vi "在image画线.vi"(10 "Image":T1, 11 "一维数组":dbl[](array[numeric])) -> (2 "Image Out":T1)   [LabVIEW 2015]
uses:
  <vilib>/vision/Image Controls.llb/IMAQ Image.ctl
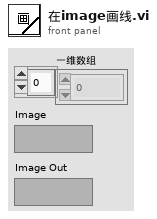
[diagram p1: front panel]
types:
  T1 = typedef "IMAQ Image.ctl" = refnum<image>
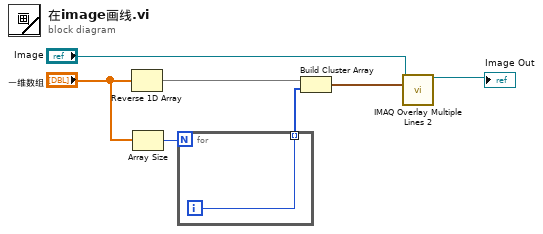
[diagram p0: block diagram]
diagram:
  n1 = Reverse 1D Array(array="一维数组") -> (reversed array=w1:dbl[])
  n2 = Array Size(array="一维数组") -> (size(s)=w6:i32)
  n3 = for {
    N: w6 -> [_]
    tunnel: [w8] -> w7 mode=indexing
    i -> [w8]
  }
  n4 = Build Cluster Array(w1, w7) -> (w5:cluster{"Numeric":dbl, i32}[])
  n5 = call "IMAQ Overlay Multiple Lines 2"("Image"="Image", "Line End Points"=w5) -> ("Image Out"=→"Image Out":T1)  [unwired: 12 in, 1 out]
